vi "Shooter.vi"   [LabVIEW 2012]
uses:
  ShooterStates.ctl
  Robot Global Data.vi
types:
  T1 = typedef "ShooterStates.ctl" = enum16{"Begin", "Spin Wheel", "Window Motor Spin", "Window Motor Wait", "Window Motor Off", "Finish"}
  T2 = typedef "WPI_MotorControlDeviceRef.ctl" = cluster{"DeviceStatus":errorcluster, "Type":enum16{"PWM", "CAN"}, "PWM":cluster{"Digital Module":T3, "PWM Channel":T4, "DeadBand":T5}, "CAN":cluster{"Device Number":u8, "Control Mode":T6, "Semaphore":T7, "Max Vout":dbl}, "Invert":bool, "TransformRef":T8, "InvTransformRef":T8}
  T3 = typedef "FPGA_TypedefDigitalModule.ctl" = enum16{"Digital Module 1", "Digital Module 2"}
  T4 = typedef "FPGA_DIOPWMChannel.ctl" = enum8{"PWM 1", "PWM 2", "PWM 3", "PWM 4", "PWM 5", "PWM 6", "PWM 7", "PWM 8", "PWM 9", "PWM 10", "Invalid"}
  T5 = typedef "WPI_PWMDeadband.ctl" = cluster{"Name":string, "maxPositivePwm":i32, "minPositivePwm":i32, "centerPwm":i32, "maxNegativePwm":i32, "minNegativePwm":i32, "angularRange":u16}
  T6 = typedef "WPI_CANJaguar_ControlMode.ctl" = enum8{"Percent VBus", "Current", "Speed", "Position", "Voltage"}
  T7 = typedef "Semaphore RefNum" = refnum<k1>
  T8 = typedef "WPI_PWMTransform_ConPane.ctl" = refnum<vi>
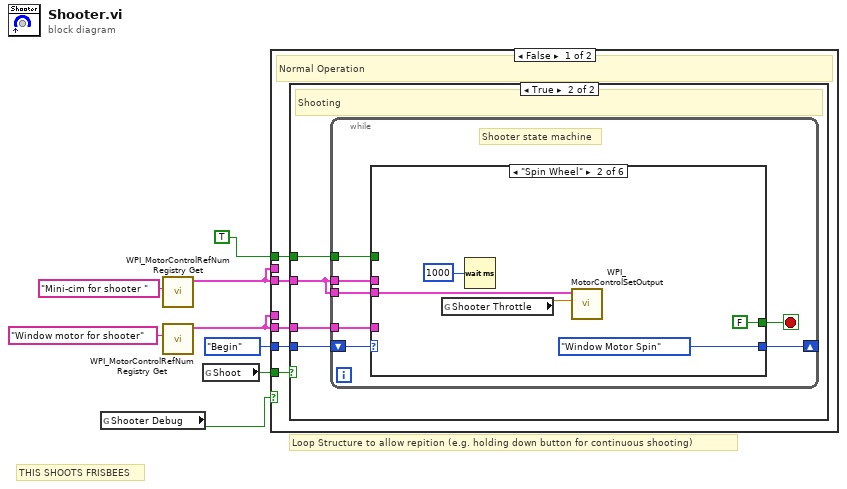
[diagram p0: block diagram]
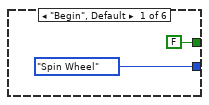
[diagram p3: hidden frame]
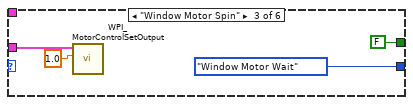
[diagram p4: hidden frame]
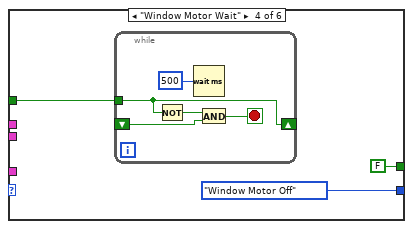
[diagram p5: hidden frame]
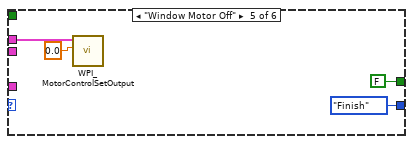
[diagram p6: hidden frame]
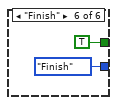
[diagram p7: hidden frame]
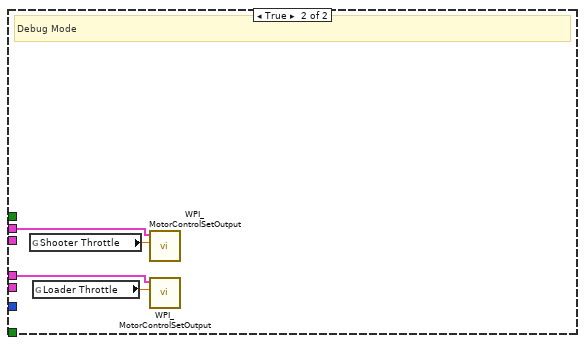
[diagram p8: hidden frame]
diagram:
  # "Loop Structure to allow repition (e.g. holding down button for continuous shooting)"
  # "THIS SHOOTS FRISBEES"
  n1 = global read "Robot Global Data.vi" "Shooter Debug"() -> (w1:bool)
  n2 = call <vilib>:"WPI_MotorControlRefNum Registry Get.vi"("refnum name"="Mini-cim for shooter ") -> ("MotorControlDevRef"=w4:T2)  [unwired: 9 in, 1 out]
  n3 = call <vilib>:"WPI_MotorControlRefNum Registry Get.vi"("refnum name"="Window motor for shooter") -> ("MotorControlDevRef"=w3:T2)  [unwired: 9 in, 1 out]
  n4 = global read "Robot Global Data.vi" "Shoot"() -> (w5:bool)
  n5 = case shown="False" w1 {
    tunnel: ShooterStates."Begin" -> [w13 _]
    tunnel: w3 -> [w12 _]
    tunnel: TRUE -> [w11 _]
    tunnel: w4 -> [w10 _]
    tunnel: w5 -> [w9 _]
    tunnel: w4 -> [_ w52]
    tunnel: w3 -> [_ w51]
    frame False {
      # "Normal Operation"
      n6 = case shown="True" w9 {
        tunnel: w13 -> [_ w17]
        tunnel: w12 -> [_ w16]
        tunnel: w11 -> [_ w15]
        tunnel: w10 -> [_ w14]
        frame False {
          # "Not Shooting"
        }
        frame True {
          # "Shooting"
          n7 = while {
            shift-right: [w23] -> _
            shift-left: w17 -> [w24]
            tunnel: w14 -> [w22]
            tunnel: w16 -> [w21]
            tunnel: w15 -> [w20]
            tunnel: w14 -> [w19]
            stop <- w18 stop-if-true
            # "Shooter state machine"
            n8 = case shown="\"Spin Wheel\"" w24 {
              tunnel: [ShooterStates."Spin Wheel" ShooterStates."Window Motor Spin" ShooterStates."Window Motor Wait" ShooterStates."Window Motor Off" ShooterStates."Finish" ShooterStates."Finish"] -> w23
              tunnel: w22 -> [_ w29 _ _ _ _]
              tunnel: w21 -> [_ _ w34 _ _ _]
              tunnel: w20 -> [_ _ _ w38 _ _]
              tunnel: w19 -> [_ _ _ _ w46 _]
              tunnel: [FALSE FALSE FALSE FALSE FALSE TRUE] -> w18
              frame "Begin", Default {
              }
              frame "Spin Wheel" {
                n9 = global read "Robot Global Data.vi" "Shooter Throttle"() -> (w30:dbl)
                n10 = Wait (ms)(milliseconds to wait=u32 1000) -> ()  [unwired: 1 out]
                n11 = call <vilib>:"WPI_MotorControlSetOutput.vi"("Output"=w30, "MotorControlDevRef"=w29) -> ()  [unwired: 7 in, 3 out]
              }
              frame "Window Motor Spin" {
                n12 = call <vilib>:"WPI_MotorControlSetOutput.vi"("Output"=1.0, "MotorControlDevRef"=w34) -> ()  [unwired: 7 in, 3 out]
              }
              frame "Window Motor Wait" {
                n13 = while {
                  shift-right: [w40] -> _
                  shift-left: _ -> [w42]
                  tunnel: w38 -> [w40]
                  stop <- w39 stop-if-true
                  n14 = Not(x=w40) -> (.not. x?=w41:bool)
                  n15 = Wait (ms)(milliseconds to wait=u32 500 ("millisecond timer value")) -> ()  [unwired: 1 out]
                  n16 = And(x=w41, y=w42) -> (x .and. y?=w39:bool)
                }
              }
              frame "Window Motor Off" {
                n17 = call <vilib>:"WPI_MotorControlSetOutput.vi"("Output"=0.0, "MotorControlDevRef"=w46) -> ()  [unwired: 7 in, 3 out]
              }
              frame "Finish" {
              }
            }
          }
        }
      }
    }
    frame True {
      # "Debug Mode"
      n18 = global read "Robot Global Data.vi" "Shooter Throttle"() -> (w53:dbl)
      n19 = global read "Robot Global Data.vi" "Loader Throttle"() -> (w50:dbl)
      n20 = call <vilib>:"WPI_MotorControlSetOutput.vi"("Output"=w53, "MotorControlDevRef"=w52) -> ()  [unwired: 7 in, 3 out]
      n21 = call <vilib>:"WPI_MotorControlSetOutput.vi"("Output"=w50, "MotorControlDevRef"=w51) -> ()  [unwired: 7 in, 3 out]
    }
  }
